vi "StartAsynchroneViAndTranslate.vi"(7 "Open Front Panel ?":bool, 8 "error in":errorcluster, 11 "viPathToStart":path) -> (0 "error out":errorcluster, 3 "vi reference":refnum<vi>)   [LabVIEW 2009]
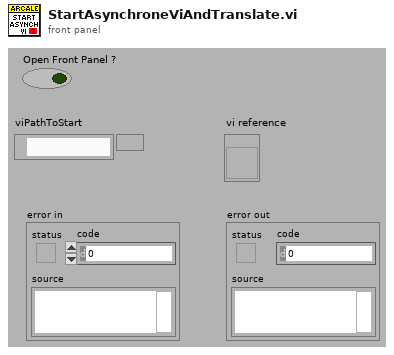
[diagram p1: front panel]
types:
  T1 = enum32{"Bad", "Idle", "Run top level", "Running"}
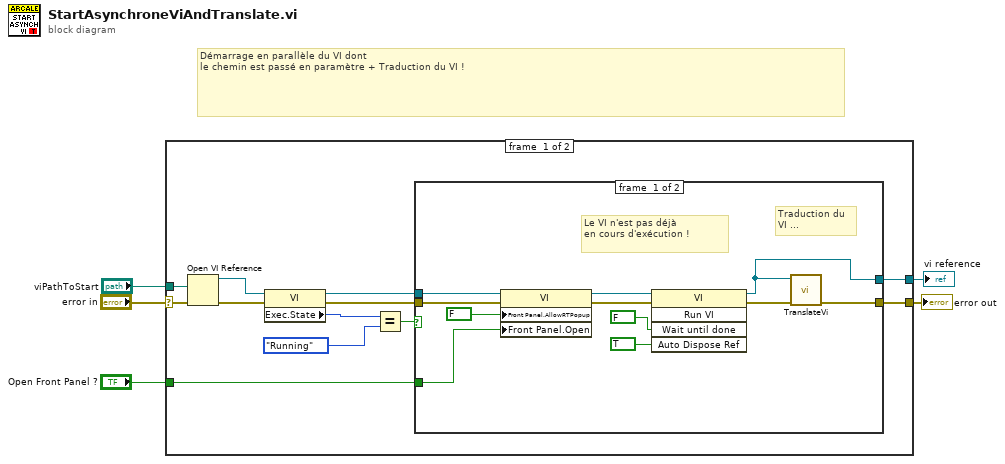
[diagram p0: block diagram]
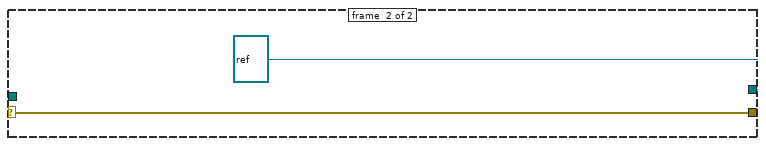
[diagram p3: hidden frame]
diagram:
  # "Démarrage en parallèle du VI dont\nle chemin est passé en paramètre + Traduction du VI !"
  n1 = case shown="No Error" "error in" {
    selector: "error in" -> [w9 w32]
    tunnel: [w6 w32] -> w5
    tunnel: [w7 refnum<vi> refnum ("vi reference")] -> w4
    tunnel: "Open Front Panel ?" -> [w17 _]
    tunnel: "viPathToStart" -> [w8 _]
    frame #0 {
      n2 = Open VI Reference(vi path=w8, error in (no error)=w9) -> (vi reference=w12:refnum<vi>, error out=w14:errorcluster)  [unwired: 1 in, 3 out]
      n3 = property class="VI"(reference=w12, error in=w14) -> (reference out=w11:refnum<vi>, error out=w13:errorcluster, "Exec.State"=w16:T1)
      n4 = Equal?(x=w16, y=T1."Running") -> (x = y?=w10:bool)
      n5 = case shown="False" w10 {
        tunnel: [w19 w30] -> w6
        tunnel: [w18 w29] -> w7
        tunnel: w13 -> [w24 w30]
        tunnel: w11 -> [w26 w29]
        tunnel: w17 -> [w21 _]
        frame #0 {
          # "Traduction du\nVI ..."
          # "Le VI n'est pas déjà\nen cours d'exécution !"
          n6 = property class="VI"(reference=w26, error in=w24, "Front Panel.AllowRTPopup"=FALSE ("Front Panel Window:Allow Runtime PopUp"), "Front Panel.Open"=w21) -> (reference out=w25:refnum<vi>, error out=w23:errorcluster)
          n7 = invoke class="VI" method="Run VI"(reference=w25, error in=w23, "Wait until done"=FALSE ("Wait Until Done"), "Auto Dispose Ref"=TRUE ("Auto Dispose Reference")) -> (reference out=w18:refnum<vi>, error out=w20:errorcluster)  [unwired: 1 in, 3 out]
          n8 = call "TranslateVi.vi"("error in (no error)"=w20, "VI ref"=w18) -> ("error out"=w19:errorcluster)  [unwired: 9 in]
        }
        frame #1 {
        }
      }
    }
    frame #1 {
    }
  }
  "error out" <- w5
  "vi reference" <- w4
